vi "GaiaReleaseDUT.vi"(8 "error in (no error)":errorcluster, 11 ".NET Refnum in":refnum<k24>) -> (0 "error out":errorcluster, 3 ".NET Refnum out":refnum<k24>)   [LabVIEW 2018]
uses:
  C:/GIT/gaialabviewclient/Gaia_LabVIEW/Resources/JOT.GaiaClient.dll
  Gaia_LabVIEW/Resources/JOT.GaiaClient.dll
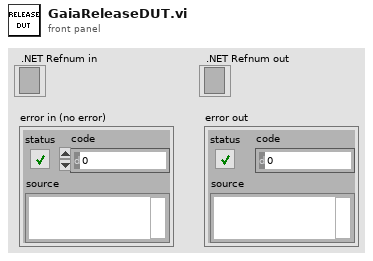
[diagram p1: front panel]
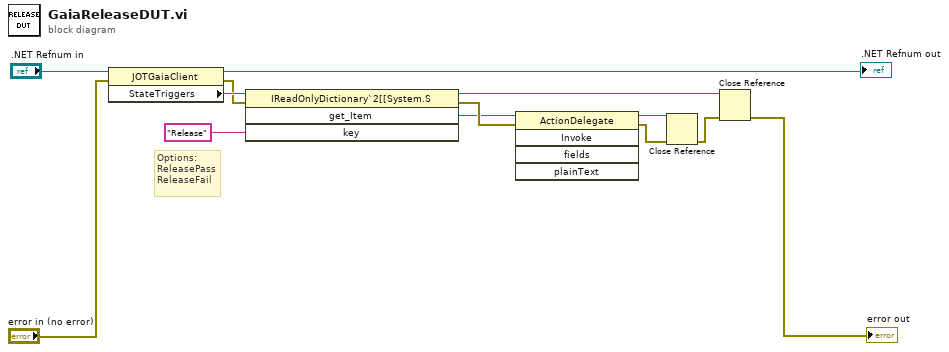
[diagram p0: block diagram]
diagram:
  # "Options:\nReleasePass\nReleaseFail"
  n1 = property class="JOTGaiaClient"(reference=".NET Refnum in", error in="error in (no error)") -> (reference out=→".NET Refnum out":refnum<k24>, error out=w5:errorcluster, "StateTriggers"=w7:refnum<k24>)
  n2 = invoke class="IReadOnlyDictionary`2[[System.S" method="get_Item"(reference=w7, error in=w5, "key"="Release") -> (reference out=w10:refnum<k24>, error out=w8:errorcluster, "get_Item"=w6:refnum<k24>)  [unwired: 1 in, 1 out]
  n3 = invoke class="ActionDelegate" method="Invoke"(reference=w6, error in=w8) -> (reference out=w9:refnum<k24>, error out=w12:errorcluster)  [unwired: 3 in, 3 out]
  n4 = Close Reference(reference=w9, error in (no error)=w12) -> (error out=w11:errorcluster)
  n5 = Close Reference(reference=w10, error in (no error)=w11) -> (error out=→"error out":errorcluster)
